vi "6514_Max_speed_2011.vi"() -> ()   [LabVIEW 2015]
panel:
  out "Data":sgl[](array[numeric])
  out "Read/s":dbl
  out "Timing":u32
  out "read buffer":string
  in  "stop":bool
  in  "VISA resource name":refnum<visa-resource-name>
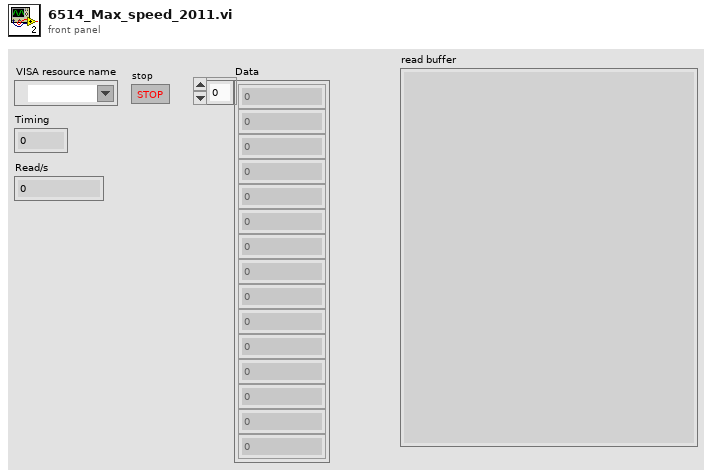
[diagram p1: front panel]
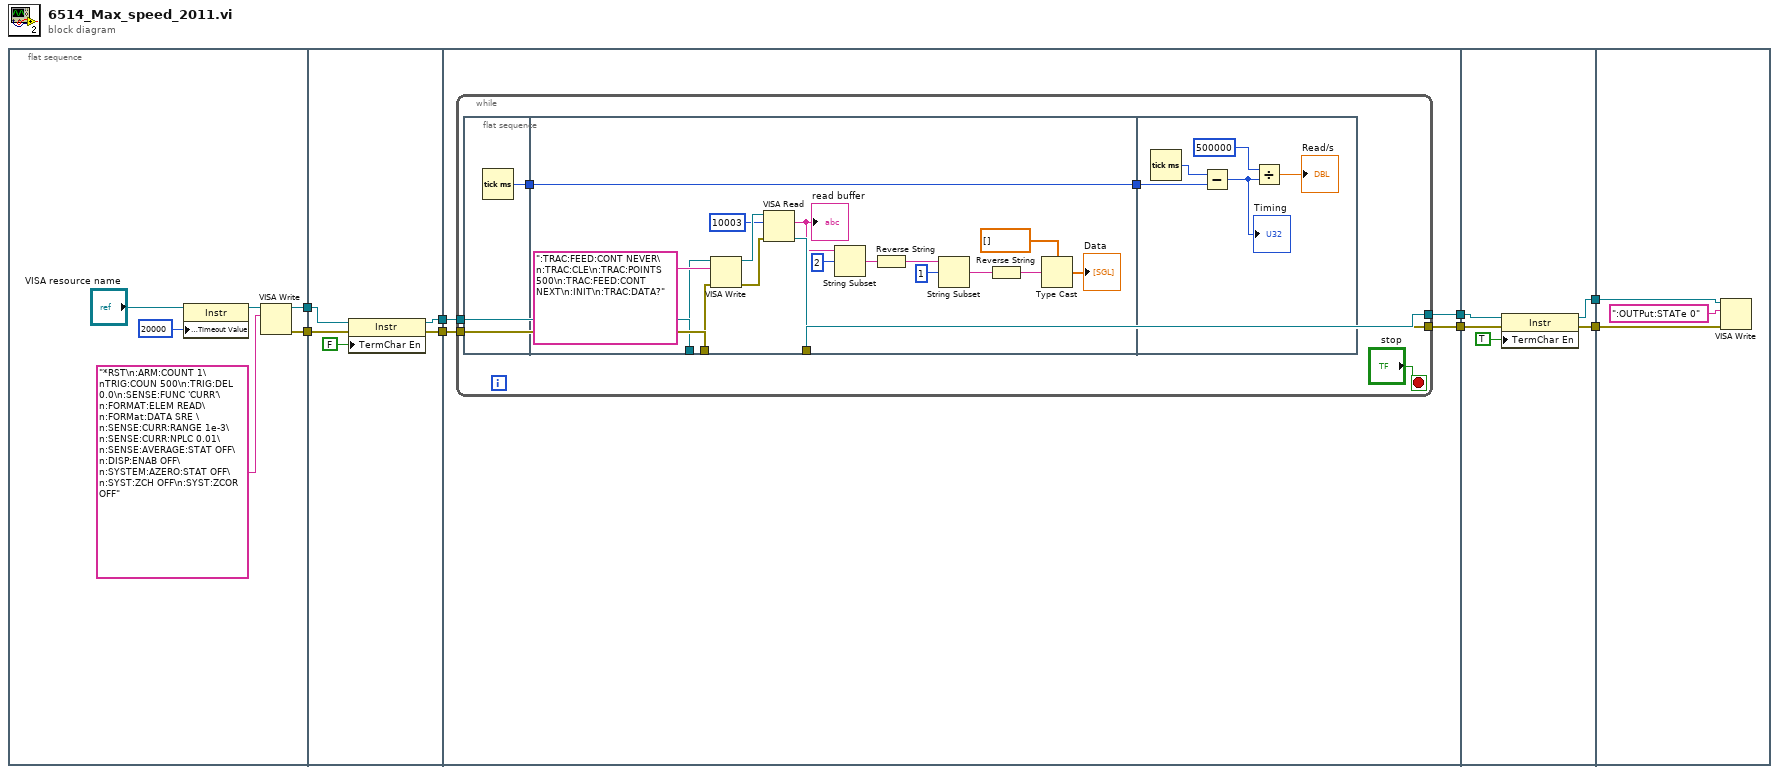
[diagram p0: block diagram]
diagram:
  n1 = flat-sequence {
    tunnel: [w10] -> w8
    tunnel: [w9] -> w6
    tunnel: w8 -> [w18]
    tunnel: [w16] -> w7
    tunnel: w6 -> [w17]
    tunnel: [w15] -> w5
    tunnel: w7 -> [w23]
    tunnel: [w22] -> w4
    tunnel: [w21] -> w2
    tunnel: w5 -> [w20]
    tunnel: w4 -> [w58]
    tunnel: [w56] -> w3
    tunnel: w2 -> [w57]
    tunnel: [w55] -> w1
    tunnel: w3 -> [w61]
    tunnel: w1 -> [w60]
    frame #0 {
      n2 = property class="Instr"(reference="VISA resource name", "General Settings:Timeout Value"=u32 20000) -> (reference out=w11:refnum<visa-resource-name>)  [unwired: 1 in, 1 out]
      n3 = VISA Write(VISA resource name=w11, write buffer="*RST\n:ARM:COUNT 1\nTRIG:COUN 500\n:TRIG:DEL 0.0\n:SENSE:FUNC 'CURR'\n:FORMAT:ELEM READ\n:FORMat:DATA SRE \n:SENSE:CURR:RANGE 1e-3\n:SENSE:CURR:NPLC 0.01\n:SENSE:AVERAGE:STAT OFF\n:DISP:ENAB OFF\n:SYSTEM:AZERO:STAT OFF\n:SYST:ZCH OFF\n:SYST:ZCOR OFF") -> (VISA resource name out=w10:refnum<visa-resource-name>, error out=w9:errorcluster)  [unwired: 1 in, 1 out]
    }
    frame #1 {
      n4 = property class="Instr"(reference=w18, error in=w17, "TermChar En"=FALSE ("Message Based Settings:Termination Character Enable")) -> (reference out=w16:refnum<visa-resource-name>, error out=w15:errorcluster)
    }
    frame #2 {
      n5 = while {
        tunnel: w23 -> [w24]
        tunnel: [w29] -> w22
        tunnel: [w27] -> w21
        tunnel: w20 -> [w26]
        stop <- "stop" stop-if-true
        n6 = flat-sequence {
          tunnel: [w31] -> w28
          tunnel: [w46] -> w29
          tunnel: [w45] -> w25
          tunnel: w28 -> [w45]
          tunnel: [w43] -> w27
          tunnel: w26 -> [w42]
          tunnel: w24 -> [w32]
          tunnel: w25 -> [w50]
          frame #0 {
            n7 = Tick Count (ms)() -> (millisecond timer value=w31:u32)
          }
          frame #1 {
            n8 = VISA Write(VISA resource name=w32, write buffer=":TRAC:FEED:CONT NEVER\n:TRAC:CLE\n:TRAC:POINTS 500\n:TRAC:FEED:CONT NEXT\n:INIT\n:TRAC:DATA?", error in (no error)=w42) -> (VISA resource name out=w48:refnum<visa-resource-name>, error out=w44:errorcluster)  [unwired: 1 out]
            n9 = VISA Read(VISA resource name=w48, byte count=u32 10003, error in (no error)=w44) -> (VISA resource name out=w46:refnum<visa-resource-name>, read buffer=w40:string, error out=w43:errorcluster)  [unwired: 1 out]
            "read buffer" <- w40
            n10 = String Subset(string=w40, offset (0)=2) -> (substring=w39:string)  [unwired: 1 in]
            n11 = Reverse String(1:w39) -> (0:w38:string)
            n12 = String Subset(string=w38, offset (0)=1) -> (substring=w36:string)  [unwired: 1 in]
            n13 = Reverse String(1:w36) -> (0:w33:string)
            n14 = Type Cast(type=sgl[] [], x=w33) -> (*(type *) &x=→"Data":sgl[])
          }
          frame #2 {
            n15 = Tick Count (ms)() -> (millisecond timer value=w51:u32)
            n16 = Subtract(x=w51, y=w50) -> (x-y=w54:u32)
            "Timing" <- w54
            n17 = Divide(x=500000, y=w54) -> (x/y=→"Read/s":dbl)
          }
        }
      }
    }
    frame #3 {
      n18 = property class="Instr"(reference=w58, error in=w57, "TermChar En"=TRUE ("Message Based Settings:Termination Character Enable")) -> (reference out=w56:refnum<visa-resource-name>, error out=w55:errorcluster)
    }
    frame #4 {
      n19 = VISA Write(VISA resource name=w61, write buffer=":OUTPut:STATe 0", error in (no error)=w60) -> ()  [unwired: 3 out]
    }
  }
